vi "Subscribe to SV.vi"(8 "error in (no error)":errorcluster, 10 "SV to subscribe to":string[](array[string]), 11 "Father of all uServices in":refnum<class "Father of all uServices.lvclass">) -> (3 "shared variable value change notification":refnum<user-event>)   [LabVIEW 2020, in "TALOS.lvlib" / "Father of all uServices.lvlib" / "Father of all uServices.lvclass"]
uses:
  Father of all uServices.lvclass
  Ancestor/Ancestor/Ancestor.lvclass/Ancestor.ctl
  Support VIs/Generate Error.vi
  FGV/Error Memory/Get Error Description.vi
  Support VIs/Get PC name.vi
  Ancestor/Ancestor/Read ID.vi
  Support VIs/Get Class Name.vi
  FGV/Error Memory/Error Memory Core.vi
  <vilib>/AdvancedString/Delimited String to 1D String Array.vi
  Support VIs/Circus Root Path.vi
  FGV/Error Memory/Error Crt Lvl checker.vi
  FGV/Error Memory/Error Memory Core.vi/40c8088d-b597-4017-91af-faa98e00292e.vi
  FGV/Error Memory/Error Memory Core.vi/d4a3ab98-063c-4e44-b43d-fbdcfe6c2be2.vi
  Support VIs/Global Memory.vi
  <vilib>/Utility/LVClass/Get LV Class Name.vi
  Support VIs/Is in Packed Library.vi
  Support VIs/TALOS Root path.vi
  Support VIs/Read CSV worksheet.vi
  Support VIs/Global Constants.vi
  <vilib>/Utility/error.llb/General Error Handler.vi
  Ancestor/Ancestor/Ancestor.lvclass
  <vilib>/Comparison/Equal/Equal Functor/Equal Functor.lvclass
  <vilib>/lvdsc/NI_DSC.lvlib
  TALOS.lvlib
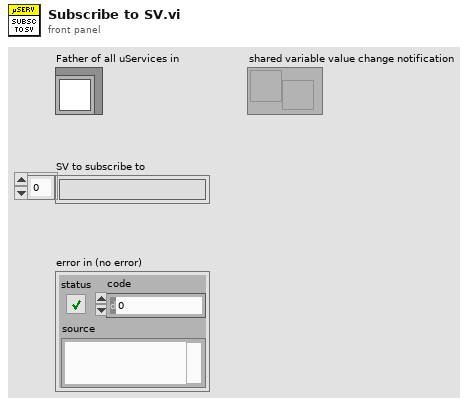
[diagram p1: front panel]
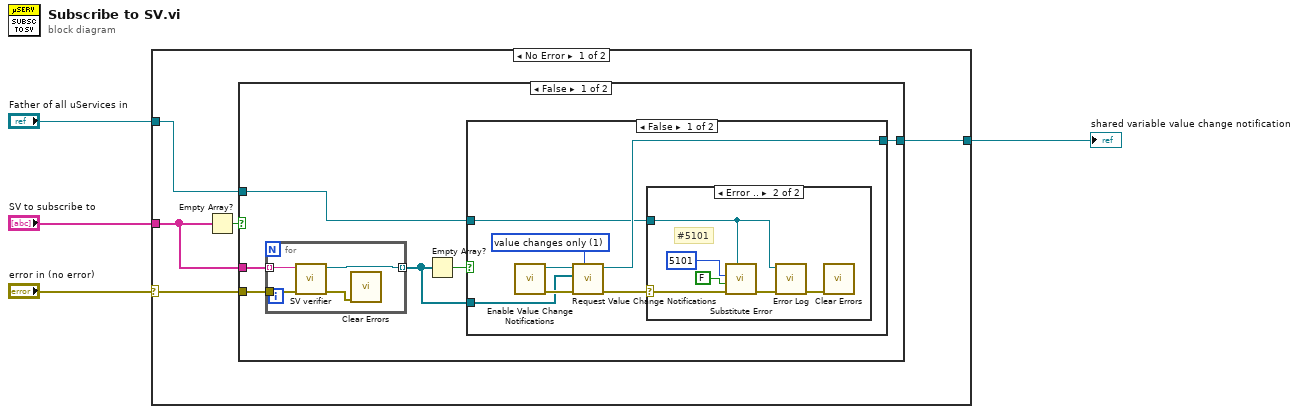
[diagram p0: block diagram]
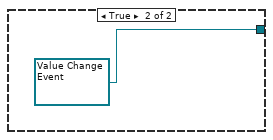
[diagram p3: hidden frame]
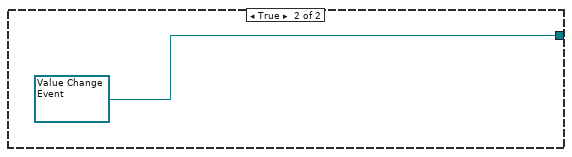
[diagram p4: hidden frame]
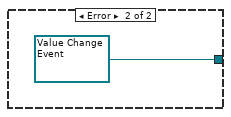
[diagram p5: hidden frame]
diagram:
  n1 = case shown="No Error" "error in (no error)" {
    selector: "error in (no error)" -> [w5 _]
    tunnel: "Father of all uServices in" -> [w9 _]
    tunnel: "SV to subscribe to" -> [w8 _]
    tunnel: [w6 refnum<user-event> refnum ("shared variable value change notification")] -> w1
    frame No Error {
      n2 = Empty Array?(array=w8) -> (empty?=w7:bool)
      n3 = case shown="False" w7 {
        tunnel: [w15 refnum<user-event> refnum ("shared variable value change notification")] -> w6
        tunnel: w5 -> [w13 _]
        tunnel: w9 -> [w14 _]
        tunnel: w8 -> [w12 _]
        frame False {
          n4 = for {
            tunnel: w12 -> [w18] mode=indexing
            tunnel: w13 -> [w19]
            tunnel: [w17] -> w11 mode=indexing
            n5 = call "SV verifier.vi"("error in (no error)"=w19, "SV name in"=w18) -> ("error out"=w16:errorcluster, "Refnum out"=w17:refnum<k21>)  [unwired: 8 in]
            n6 = call <vilib>:"Clear Errors.vi"("error in (no error)"=w16) -> ()  [unwired: 5 in, 2 out]
          }
          n7 = Empty Array?(array=w11) -> (empty?=w10:bool)
          n8 = case shown="False" w10 {
            tunnel: [w26 refnum<user-event> refnum ("shared variable value change notification")] -> w15
            tunnel: w14 -> [w22 _]
            tunnel: w11 -> [w20 _]
            frame False {
              w23 = u16 1 items=["all changes", "value changes only"] ("request changes (all changes)")
              n9 = call <vilib>:"Enable Value Change Notifications.vi"() -> ("error out"=w25:errorcluster, "shared variable value change notification"=w24:refnum<user-event>)  [unwired: 10 in]
              n10 = call <vilib>:"Request Value Change Notifications.vi"("request changes (all changes)"=w23, "error in (no error)"=w25, "shared variables"=w20, "notification refnum"=w24) -> ("error out"=w21:errorcluster, "shared variable value change notification"=w26:refnum<user-event>)  [unwired: 5 in, 1 out]
              n11 = case shown="Error .." w21 {
                selector: w21 -> [_ w32]
                tunnel: w22 -> [_ w27]
                frame No Error {
                }
                frame Error {
                  # "#5101"
                  n12 = call "Substitute Error.vi"("LabVIEW Object"=w27, "error in (no error)"=w32, "Error/Warning"=FALSE, "Error Code"=5101) -> ("error out"=w29:errorcluster)  [unwired: 7 in]
                  n13 = call "Error Log.vi"("error in (no error)"=w29, "Object in"=w27) -> ("error out"=w28:errorcluster)  [unwired: 9 in]
                  n14 = call <vilib>:"Clear Errors.vi"("error in (no error)"=w28) -> ()  [unwired: 5 in, 2 out]
                }
              }
            }
            frame True {
            }
          }
        }
        frame True {
        }
      }
    }
    frame Error {
    }
  }
  "shared variable value change notification" <- w1
